vi "TstBldr_StimulusProfile.vi"(0 "Engine reference":refnum<k7>, 1 "Paths":T3, 2 "First call?":bool=TRUE, 5 "Sequence File Ref":refnum<k7>, 7 "VeriStand version info":T1, 9 "Step Name":string="Run Stim Profile", 11 "error in":errorcluster, 12 "Sequence index":i32, 13 "Condition Run?":bool, 14 "Requirement":string) -> (3 "First call? out":bool, 4 "Engine reference (out)":refnum<k7>, 6 "Sequence File Ref(out)":refnum<k7>, 10 "Sequence index (out)":i32, 15 "error out":errorcluster)   [LabVIEW 2010]
doc: "This VI adds the TestStand steps for running a Stimulus Profile and wait until it is done"
uses:
  FilePaths.ctl
  SeqBuilder/Ctls/dotNetAssemblyInfo.ctl
  SeqBuilder/Ctls/VSModuleTokens.ctl
  vs_RunStimProfSteps.ctl
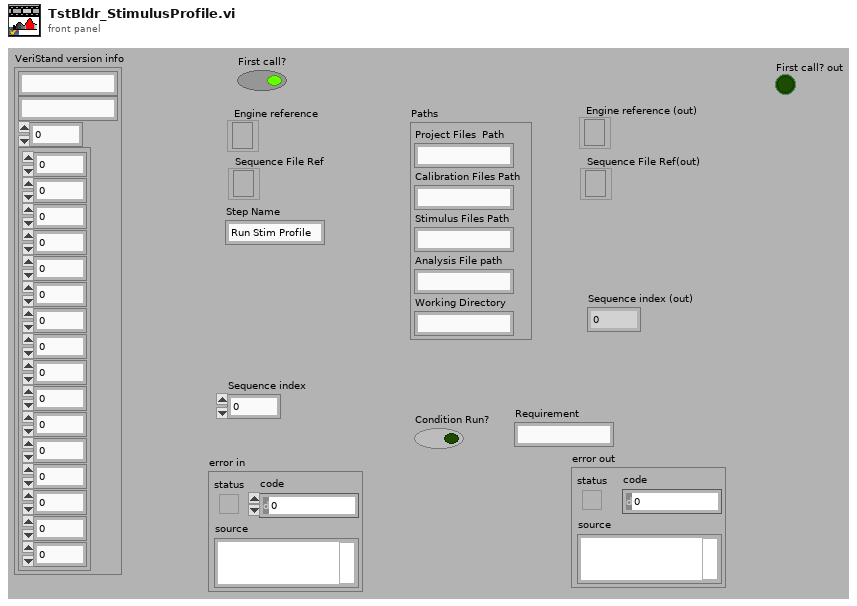
[diagram p1: front panel]
types:
  T1 = typedef "dotNetAssemblyInfo.ctl" = cluster{"VeriStand.exe Path":string, "Assembly":string, "Constructor Token":i32, "Module Token":T2}
  T2 = typedef "VSModuleTokens.ctl" = cluster{"GetIWorkspaceToken":i32, "GetIStimulusToken":i32, "GetIModelManagerToken":i32, "GetIProjectToken":i32, "RunProjectToken":i32, "CloseProjectToken":i32, "RunWorkspaceToken":i32, "StopWorkspaceToken":i32, "SetSingleChannelToken":i32, "SetMultipleParametersToken":i32, "RunStimulusToken":i32, "GetStimulusStateToken":i32, "Open WorkspaceToken":i32, "DeployToken":i32, "UndeployToken":i32, "QuitToken":i32}
  T3 = typedef "FilePaths.ctl" = cluster{"Project Files  Path":string, "Calibration Files Path":string, "Stimulus Files Path":string, "Analysis File path":string, "Working Directory":string}
  T4 = typedef "vs_RunStimProfSteps.ctl" = enum16{"Call Profile", "Wait", "Do While", "Check Stimuls State", "Wait1", "End", "Get TDMs file name", "Quit Loop"}
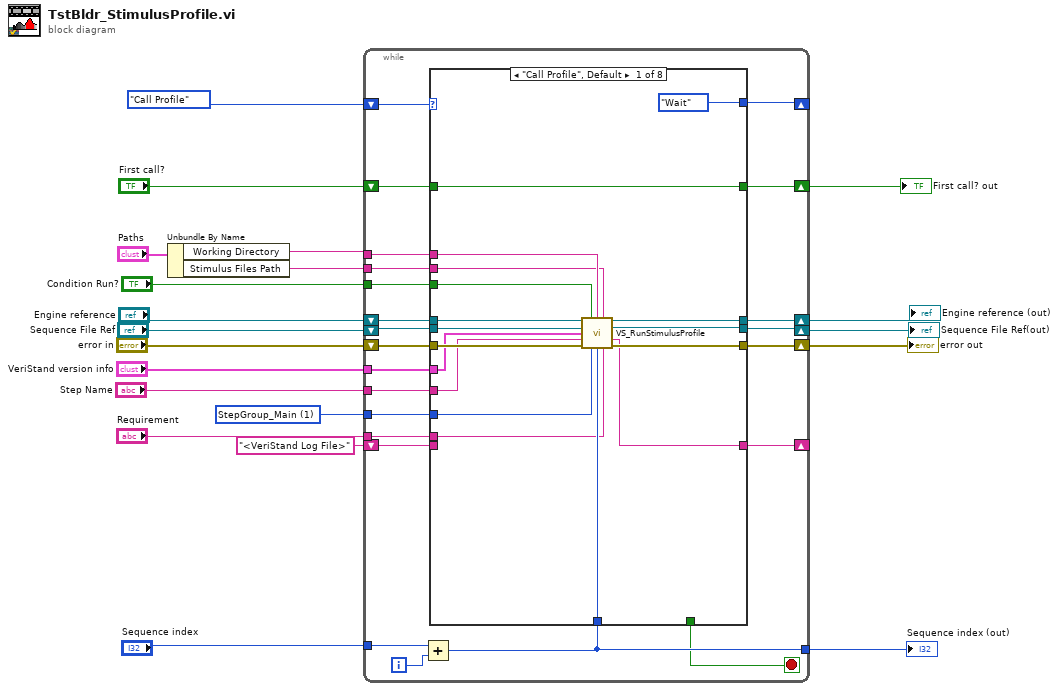
[diagram p0: block diagram]
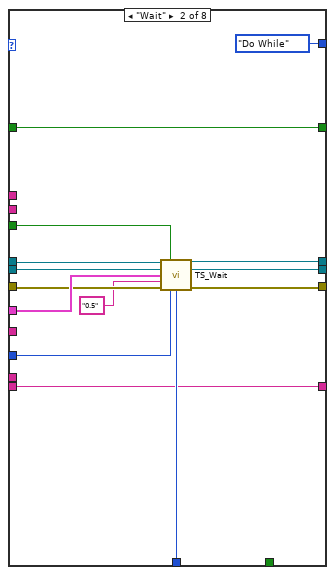
[diagram p2: hidden frame]
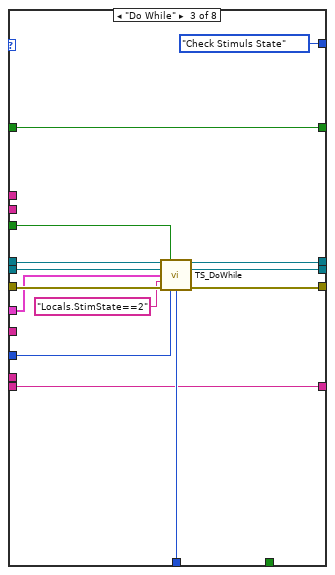
[diagram p3: hidden frame]
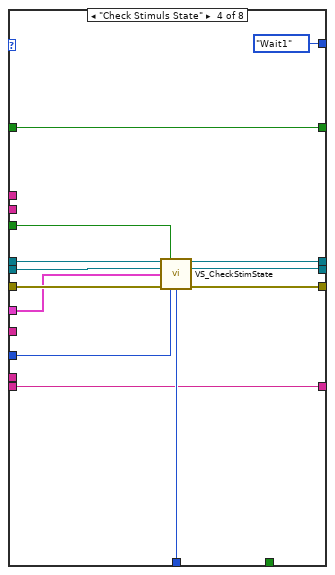
[diagram p4: hidden frame]
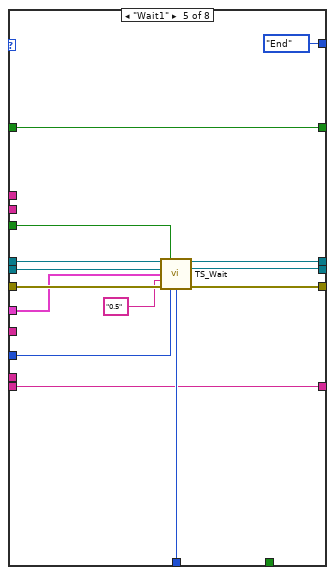
[diagram p5: hidden frame]
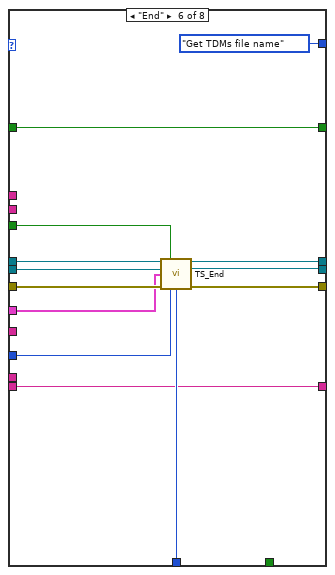
[diagram p6: hidden frame]
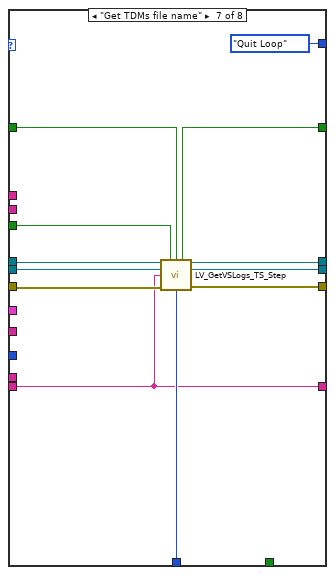
[diagram p7: hidden frame]
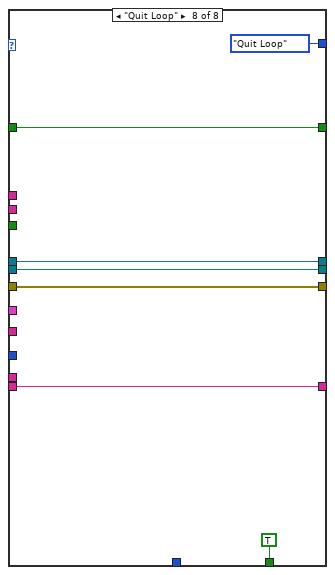
[diagram p8: hidden frame]
diagram:
  w5 = 1 items=["StepGroup_Setup", "StepGroup_Main", "StepGroup_Cleanup"] ("Step Group")
  n1 = Unbundle By Name("Paths") -> ("Working Directory"=w2:string, "Stimulus Files Path"=w1:string)
  n2 = while {
    tunnel: w2 -> [w38]
    shift-right: [w41] -> w19
    shift-left: "Sequence File Ref" -> [w42]
    shift-right: [w35] -> w18
    shift-left: "error in" -> [w39]
    shift-right: [w26] -> _
    shift-left: vs_RunStimProfSteps."Call Profile" ("Enum") -> [w43]
    tunnel: "Requirement" -> [w37]
    shift-right: [w27] -> w12
    shift-left: "First call?" -> [w36]
    tunnel: "VeriStand version info" -> [w34]
    tunnel: "Step Name" -> [w33]
    tunnel: "Sequence index" -> [w31]
    tunnel: [w30] -> w8
    shift-right: [w29] -> w7
    shift-left: "Engine reference" -> [w40]
    tunnel: "Condition Run?" -> [w28]
    tunnel: w5 -> [w25]
    shift-right: [w23] -> _
    shift-left: "<VeriStand Log File>" ("VS Log file") -> [w22]
    tunnel: w1 -> [w21]
    i -> [w32]
    stop <- w24 stop-if-true
    n3 = Add(x=w31, y=w32) -> (x+y=w30:i32)
    n4 = case shown="\"Call Profile\", Default" w43 {
      tunnel: w42 -> [w53 w73 w86 w97 w111 w122 w132 w144]
      tunnel: [w52 w65 w84 w95 w109 w124 w133 w144] -> w41
      tunnel: w40 -> [w55 w74 w87 w98 w112 w123 w139 w145]
      tunnel: w39 -> [w60 w71 w82 w99 w115 w127 w138 w143]
      tunnel: w38 -> [w49 _ _ _ _ _ _ _]
      tunnel: w37 -> [w50 _ _ _ _ _ _ _]
      tunnel: w36 -> [w48 w62 w77 w91 w104 w117 w131 w146]
      tunnel: [w59 w66 w83 w100 w114 w126 w136 w143] -> w35
      tunnel: w34 -> [w58 w72 w81 w94 w107 w121 _ _]
      tunnel: w33 -> [w57 _ _ _ _ _ _ _]
      tunnel: w30 -> [w56 w67 w88 w101 w113 w128 w137 _]
      tunnel: [w54 w64 w85 w96 w110 w125 w134 w145] -> w29
      tunnel: w28 -> [w51 w69 w78 w92 w108 w120 w135 _]
      tunnel: [w48 w62 w77 w91 w104 w117 w130 w146] -> w27
      tunnel: [vs_RunStimProfSteps."Wait" ("Enum") vs_RunStimProfSteps."Do While" ("Enum") vs_RunStimProfSteps."Check Stimuls State" ("Enum") vs_RunStimProfSteps."Wait1" ("Enum") vs_RunStimProfSteps."End" ("Enum") vs_RunStimProfSteps."Get TDMs file name" ("Enum") vs_RunStimProfSteps."Quit Loop" ("Enum") vs_RunStimProfSteps."Quit Loop" ("Enum")] -> w26
      tunnel: w25 -> [w46 w68 w79 w93 w105 w119 _ _]
      tunnel: [_ _ _ _ _ _ _ TRUE] -> w24
      tunnel: [w45 w61 w75 w89 w102 w116 w129 w141] -> w23
      tunnel: w22 -> [_ w61 w75 w89 w102 w116 w129 w141]
      tunnel: w21 -> [w44 _ _ _ _ _ _ _]
      frame "Call Profile", Default {
        n5 = call "VS_RunStimulusProfile.vi"("Engine Reference(in)"=w55, "Condition Run?"=w51, "Working Directory"=w49, "Stim Profile path"=w44, "Sequence File Ref(in)"=w53, "VeriStand version info"=w58, "Stim profile"=w57, "error in"=w60, "Step Group"=w46, "Step Index"=w56, "Requirement"=w50) -> ("Engine reference(out)"=w54:refnum<k7>, "Sequence File Ref(out)"=w52:refnum<k7>, "VS Log file"=w45:string, "error out"=w59:errorcluster)  [unwired: 1 out]
      }
      frame "Wait" {
        n6 = call "TS_Wait.vi"("Engine Reference(in)"=w74, "Condition Run?"=w69, "Sequence File Ref(in)"=w73, "VeriStand version info"=w72, "Time to Wait"="0.5" ("newValue"), "error in"=w71, "Step Group"=w68, "index"=w67) -> ("Engine reference(out)"=w64:refnum<k7>, "Sequence File Ref(out)"=w65:refnum<k7>, "error out"=w66:errorcluster)  [unwired: 4 in, 1 out]
      }
      frame "Do While" {
        n7 = call "TS_DoWhile.vi"("Engine Reference(in)"=w87, "Condition Run?"=w78, "Sequence File Ref(in)"=w86, "VeriStand version info"=w81, "Condition"="Locals.StimState==2" ("newValue"), "error in"=w82, "Step Group"=w79, "index"=w88) -> ("Engine reference(out)"=w85:refnum<k7>, "Sequence File Ref(out)"=w84:refnum<k7>, "error out"=w83:errorcluster)  [unwired: 4 in, 1 out]
      }
      frame "Check Stimuls State" {
        n8 = call "VS_CheckStimState.vi"("Engine Reference(in)"=w98, "Condition Run?"=w92, "Sequence File Ref(in)"=w97, "VeriStand version info"=w94, "error in"=w99, "Step Group"=w93, "Step Index"=w101) -> ("Engine reference(out)"=w96:refnum<k7>, "Sequence File Ref(out)"=w95:refnum<k7>, "error out"=w100:errorcluster)  [unwired: 5 in, 1 out]
      }
      frame "Wait1" {
        n9 = call "TS_Wait.vi"("Engine Reference(in)"=w112, "Condition Run?"=w108, "Sequence File Ref(in)"=w111, "VeriStand version info"=w107, "Time to Wait"="0.5" ("newValue"), "error in"=w115, "Step Group"=w105, "index"=w113) -> ("Engine reference(out)"=w110:refnum<k7>, "Sequence File Ref(out)"=w109:refnum<k7>, "error out"=w114:errorcluster)  [unwired: 4 in, 1 out]
      }
      frame "End" {
        n10 = call "TS_End.vi"("Engine Reference(in)"=w123, "Condition Run?"=w120, "Sequence File Ref(in)"=w122, "VeriStand version info"=w121, "error in"=w127, "Step Group"=w119, "index"=w128) -> ("Engine reference(out)"=w125:refnum<k7>, "Sequence File Ref(out)"=w124:refnum<k7>, "error out"=w126:errorcluster)  [unwired: 5 in, 1 out]
      }
      frame "Get TDMs file name" {
        n11 = call "LV_GetVSLogs_TS_Step.vi"("Engine Reference"=w139, "Condition Run?"=w135, "First call"=w131, "Sequence File Ref"=w132, "Logs Folder"=w129, "error in"=w138, "index"=w137) -> ("First call out"=w130:bool, "Engine reference(out)"=w134:refnum<k7>, "Sequence File Ref(out)"=w133:refnum<k7>, "error out"=w136:errorcluster)  [unwired: 5 in]
      }
      frame "Quit Loop" {
      }
    }
  }
  "Sequence File Ref(out)" <- w19
  "error out" <- w18
  "Engine reference (out)" <- w7
  "Sequence index (out)" <- w8
  "First call? out" <- w12
